vi "programa2.vi"() -> ()   [LabVIEW 2011]
panel:
  out "Alarma 2":bool
  out "Alarma":bool
  out "Valor Termperatura":dbl
  out "Temperatura":i32(slide) scale=0.0..60.0
  # "Encender la alarma cuando la temperatura\nsea mayor a 40 grados."
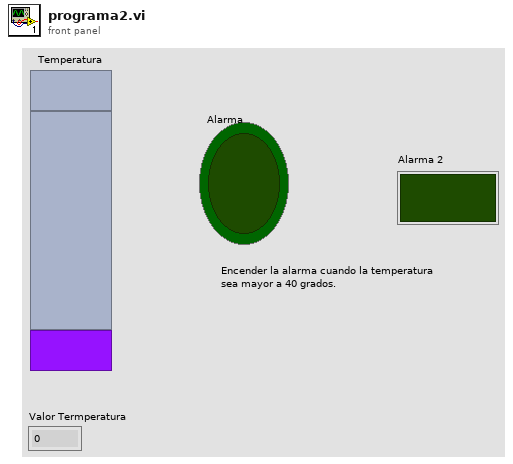
[diagram p1: front panel]
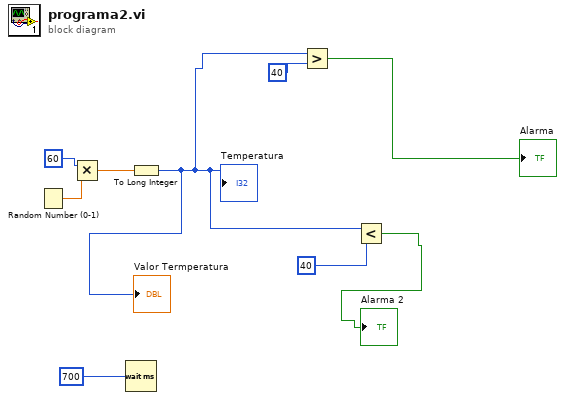
[diagram p0: block diagram]
diagram:
  n1 = Random Number (0-1)() -> (number: 0 to 1=w8:dbl)
  n2 = Multiply(x=60, y=w8) -> (x*y=w7:dbl)
  n3 = Wait (ms)(milliseconds to wait=700) -> ()  [unwired: 1 out]
  n4 = To Long Integer(number=w7) -> (32bit integer=w2:i32)
  "Temperatura" <- w2
  "Valor Termperatura" <- w2
  n5 = Greater?(x=w2, y=40) -> (0:→"Alarma":bool)
  n6 = Less?(x=w2, y=40) -> (x < y?=→"Alarma 2":bool)
